vi "LINX-Main.vi"() -> ()   [LabVIEW 2019]
doc: "This example demonstrates how to write N channels of digital ouput from a LINX device."
uses:
  <vilib>/MakerHub/LINX/Public/Peripherals/Digital/Digital Write 1 Chan.vi
  <vilib>/MakerHub/LINX/Public/Peripherals/Digital/Digital Write N Chans.vi
  <vilib>/MakerHub/LINX/Private/Local IO/LinxDigitalWrite.vi
  <vilib>/MakerHub/LINX/Public/Utilities/Check Channel.vi
  <vilib>/MakerHub/LINX/Public/Utilities/Open Serial.vi
  <vilib>/MakerHub/LINX/Private/Utilties/Generate Error.vi
  <vilib>/MakerHub/LINX/LMH-LINX.lvlib
  <vilib>/Analysis/NI_AALBase.lvlib
panel:
  out "Elapsed Time (s)":dbl
  in  "Reset":bool
  in  "Time Target (s)":dbl=1.0
  in  "Dial":dbl(knob)=500.0 min=400.0 max=2000.0 step=100.0 scale=400.0..2000.0
  in  "Enable":bool
  in  "Direction":bool
  in  "Stop Button":bool
  in  "Serial Port":refnum<visa-resource-name>
  # "Serial Port"
  # "Controls"
  # "Simple Step Motor Driver\n\nThis simple program controls a step motor (hopefully)."
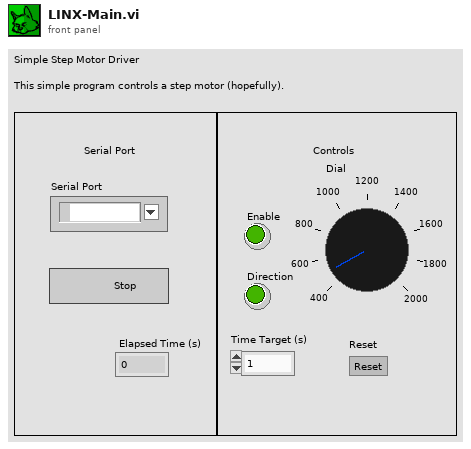
[diagram p1: front panel]
types:
  T1 = typedef "LMH-LINX.lvlib/LINX Ref.ctl" = cluster{"IO":T2, "Interface":T3, "LINX Device Config":T4}
  T2 = typedef "LMH-LINX.lvlib/Platform.ctl" = enum16{"Remote", "Local"}
  T3 = typedef "LMH-LINX.lvlib/Interface.ctl" = enum16{"Serial", "TCP"}
  T4 = typedef "LMH-LINX.lvlib/Device.lvlib/LINX Device Config.ctl" = cluster{"Interface":T3, "COM Port":refnum<visa-resource-name>, "TCP Configuration":T5, "Device Family":u8, "Device ID":u8, "Device Name":string, "TCP Ref":refnum<k5>, "Channels":T6}
  T5 = typedef "LMH-LINX.lvlib/Device.lvlib/TCP Config.ctl" = cluster{"IP Address":string, "Port":u16}
  T6 = typedef "LMH-LINX.lvlib/Channels.ctl" = cluster{"DI":u8[], "DO":u8[], "AI":u8[], "AO":u8[], "PWM":u8[], "QE":u8[], "UART":u8[], "I2C 2":u8[], "SPI":u8[], "CAN":u8[], "Servo":u8[], "AI Ref (V)":dbl, "AI Resolution (Bits)":u8, "AO Ref (V)":dbl, "AO Resolution (Bits)":u8}
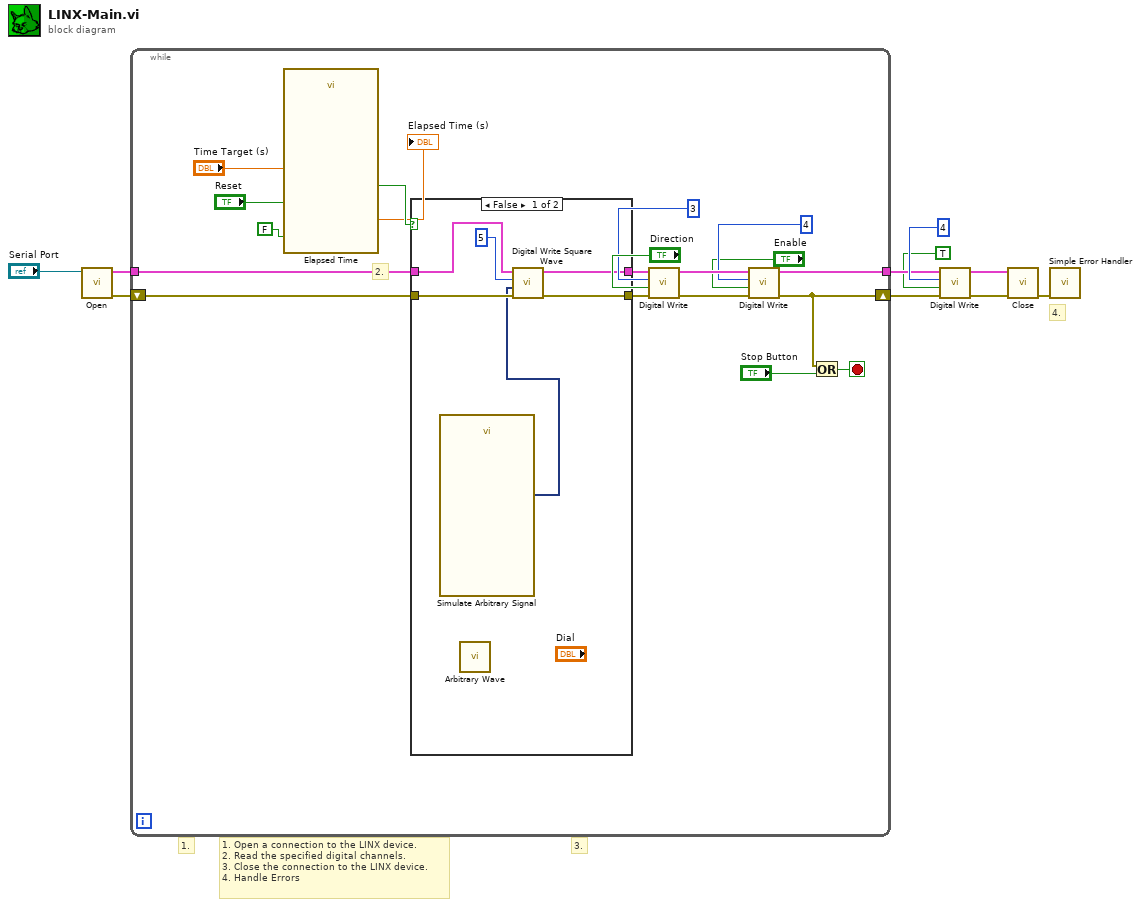
[diagram p0: block diagram]
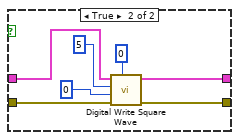
[diagram p2: hidden frame]
diagram:
  # "1. Open a connection to the LINX device.\n2. Read the specified digital channels.\n3. Close the connection to the LINX device.\n4. Handle Errors"
  # "4."
  # "3."
  # "1."
  n1 = call-poly <vilib>:"Open.vi"("Serial Port"="Serial Port") -> ("Error Out"=w9:errorcluster, "LINX Resource"=w10:T1)  [unwired: 8 in, 1 out]
  n2 = while {
    tunnel: w10 -> [w22]
    shift-right: [w26] -> w4
    shift-left: w9 -> [w20]
    tunnel: [w28] -> w5
    stop <- w15 stop-if-true
    # "2."
    n3 = call "Elapsed Time"("Time Target (s)"="Time Target (s)", "Reset"="Reset", "Auto Reset"=FALSE) -> ("Elapsed Time (s)"=→"Elapsed Time (s)":dbl, "Time has Elapsed"=w13:bool)  [unwired: 9 in, 6 out]
    n4 = case shown="False" w13 {
      tunnel: w22 -> [w34 w41]
      tunnel: [w33 w40] -> w21
      tunnel: w20 -> [w32 w39]
      tunnel: [w31 w38] -> w19
      frame False {
        n5 = call "Simulate Arbitrary Signal"() -> ("Signal"=w30:dynamicdata)  [unwired: 9 in, 2 out]
        n6 = call <vilib>:"Arbitrary Wave.vi"() -> ()  [unwired: 7 in, 3 out]
        n7 = call <vilib>:"Digital Write Square Wave.vi"("Error In"=w32, "Frequency (Hz)"=w30, "Channel"=u8 5 ("PWM Channel"), "LINX Resource"=w34) -> ("Error Out"=w31:errorcluster, "LINX Resource"=w33:T1)  [unwired: 6 in]
      }
      frame True {
        n8 = call <vilib>:"Digital Write Square Wave.vi"("Duration (ms)"=u32 0, "Error In"=w39, "Frequency (Hz)"=u32 0, "Channel"=u8 5 ("PWM Channel"), "LINX Resource"=w41) -> ("Error Out"=w38:errorcluster, "LINX Resource"=w40:T1)  [unwired: 5 in]
      }
    }
    n9 = call-poly <vilib>:"Digital Write.vi"("Error In"=w19, "Output Value"="Direction", "DO Channel"=u8 3, "LINX Resource"=w21) -> ("Error Out"=w27:errorcluster, "LINX Resource"=w29:T1)  [unwired: 6 in]
    n10 = call-poly <vilib>:"Digital Write.vi"("Error In"=w27, "Output Value"="Enable", "DO Channel"=u8 4, "LINX Resource"=w29) -> ("Error Out"=w26:errorcluster, "LINX Resource"=w28:T1)  [unwired: 6 in]
    n11 = Or(x=w26, y="Stop Button") -> (x .or. y?=w15:bool)
  }
  n12 = call-poly <vilib>:"Digital Write.vi"("Error In"=w4, "Output Value"=TRUE, "DO Channel"=u8 4, "LINX Resource"=w5) -> ("Error Out"=w3:errorcluster, "LINX Resource"=w2:T1)  [unwired: 6 in]
  n13 = call <vilib>:"Close.vi"("Error In"=w3, "LINX Resource"=w2) -> ("Error Out"=w7:errorcluster)  [unwired: 9 in]
  n14 = call <vilib>:"Simple Error Handler.vi"("error in (no error)"=w7) -> ()  [unwired: 4 in, 5 out]
